vi "SyncWindow.vi"(8 "No Error":errorcluster, 11 "Window [SDL_Window *]":i64 format="%.0x") -> (0 "Error Out":errorcluster, 3 "Timeout?":bool)   [LabVIEW 2026, in "SDL3.lvlib" / "Video.lvlib"]
doc: "<B>Summary</B>\nBlock until any pending window state is finalized.\n\n<B>Remarks</B>\nOn asynchronous windowing systems, this acts as a synchronization barrier for pending window state. It will attempt to wait until any pending window state has been applied and is guaranteed to return within finite time. Note that for how long it can potentially block depends on the underlying window system, as window state changes may involve somewhat lengthy animations that must complete before the window is in its final requested state.\n\nOn windowing systems where changes are immediate, this does nothing."
uses:
  Video.lvlib
  Lib/SDL3.dll
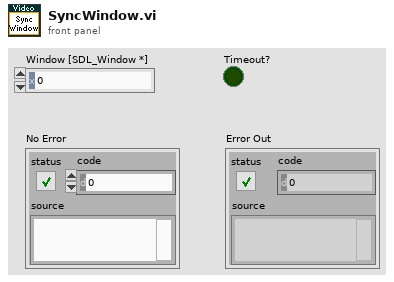
[diagram p1: front panel]
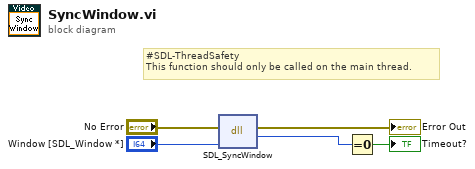
[diagram p0: block diagram]
diagram:
  # "#SDL-ThreadSafety\nThis function should only be called on the main thread."
  n1 = dll-call lib="C:/Users/saukko/Dev/LV-SDL3/Sources/SDL3/Lib/SDL3.*" fn="SDL_SyncWindow"(error in="No Error", "window"="Window [SDL_Window *]") -> (error out=→"Error Out":errorcluster, "return type"=w2:i32)  [unwired: 3 in, 1 out]
  n2 = Equal To 0?(x=w2) -> (x = 0?=→"Timeout?":bool)
